vi "parse -- check for exact match.vi"(9 "offset past match":i32, 10 "after match":string, 11 "before match":string) -> (0 "exact match":bool)   [LabVIEW 2015]
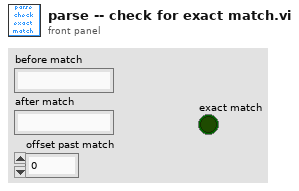
[diagram p1: front panel]
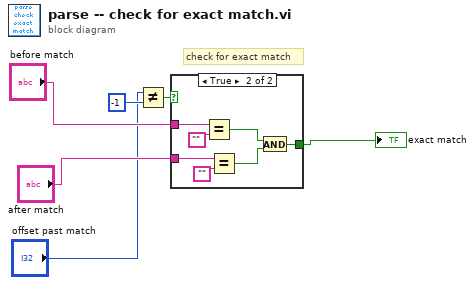
[diagram p0: block diagram]
diagram:
  # "check for exact match"
  n1 = Not Equal?(x="offset past match", y=-1) -> (x != y?=w5:bool)
  n2 = case shown="True" w5 {
    selector: w5 -> [w7 _]
    tunnel: "after match" -> [_ w13]
    tunnel: "before match" -> [_ w8]
    tunnel: [w7 w9] -> w1
    frame False {
    }
    frame True {
      n3 = Equal?(x=w8, y="") -> (x = y?=w10:bool)
      n4 = Equal?(x=w13, y="") -> (x = y?=w11:bool)
      n5 = And(x=w10, y=w11) -> (x .and. y?=w9:bool)
    }
  }
  "exact match" <- w1
